vi "Benchmark - Delta Time.vi"() -> ()   [LabVIEW 2020, in "Utility.lvlib"]
uses:
  Utility.lvlib
  <vilib>/Analysis/NI_AALBase.lvlib
  Benchmark/Benchmark.lvlib
  8ca8b4a3-a15b-4534-87bf-3f66f767895e.vi
panel:
  out "Std Dev":dbl format="%.1p"
  out "Mean":dbl format="%.1p"
  out "Histogram Graph":T1(graph)
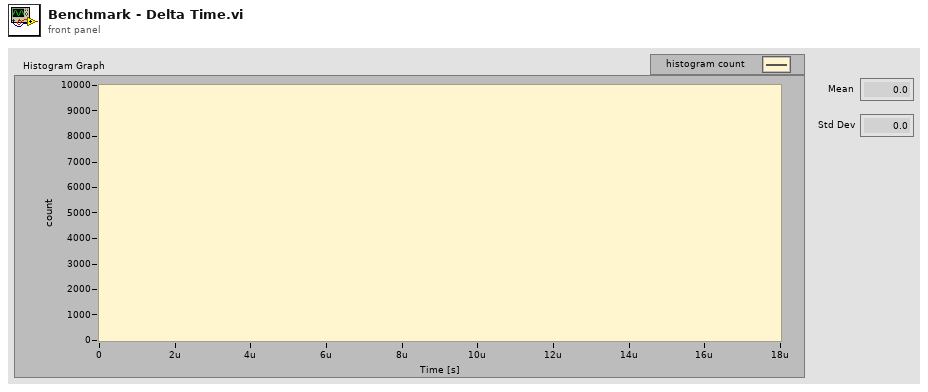
[diagram p1: front panel]
types:
  T1 = cluster{"X Values":dbl[], "Histogram: h(x)":i32[]}
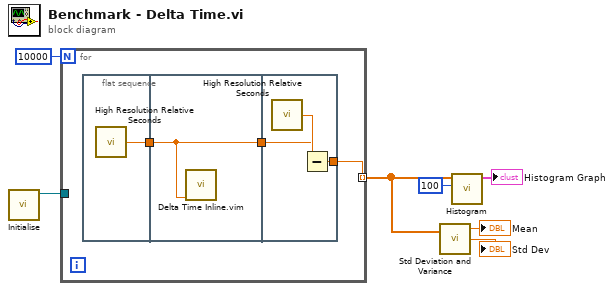
[diagram p0: block diagram]
diagram:
  n1 = call "Initialise.vi"() -> ("Scene out"=w4:refnum<class "Scene.lvclass">)  [unwired: 10 in, 1 out]
  n2 = for {
    N: 10000 -> [_]
    tunnel: w4 -> [_]
    tunnel: [w8] -> w3 mode=indexing
    n3 = flat-sequence {
      tunnel: [w11] -> w10
      tunnel: w10 -> [w12]
      tunnel: [w12] -> w9
      tunnel: w9 -> [w14]
      tunnel: [w13] -> w8
      frame #0 {
        n4 = call <vilib>:"High Resolution Relative Seconds.vi"() -> ("relative seconds"=w11:dbl)
      }
      frame #1 {
        n5 = call "Delta Time Inline.vim"("value in"=w12) -> ()  [unwired: 8 in, 3 out]
      }
      frame #2 {
        n6 = call <vilib>:"High Resolution Relative Seconds.vi"() -> ("relative seconds"=w15:dbl)
        n7 = Subtract(x=w15, y=w14) -> (x-y=w13:dbl)
      }
    }
  }
  n8 = call <vilib>:"Std Deviation and Variance.vi"("X"=w3) -> ("mean"=→"Mean":dbl, "standard deviation"=→"Std Dev":dbl)  [unwired: 1 in, 1 out]
  n9 = call <vilib>:"Histogram.vi"("intervals"=100, "X"=w3) -> ("Histogram Graph"=→"Histogram Graph":T1)  [unwired: 6 in, 3 out]
